vi "Look up Running Measurement Queue .vi"(7 "error in (no error)":errorcluster, 9 "Measurement Name.Harware()":string, 10 "Mag Lab Measure Controller in":refnum<class "Mag Lab Measure Controller.lvclass">) -> (0 "error out":errorcluster, 1 "Measurement Queue":refnum<class "Message Enqueuer.lvclass">, 2 "Found?":bool, 3 "Mag Lab Measure Controller out":refnum<class "Mag Lab Measure Controller.lvclass">)   [LabVIEW 2015, in "Mag Lab Measure Controller.lvclass"]
uses:
  Mag Lab Measure Controller.lvclass
  <vilib>/ActorFramework/Message Enqueuer/Message Enqueuer.lvclass
  Mag Lab Measure Controller.lvclass/Mag Lab Measure Controller.ctl
panel:
  in  "Self Enqueuer":refnum<class "Message Enqueuer.lvclass">
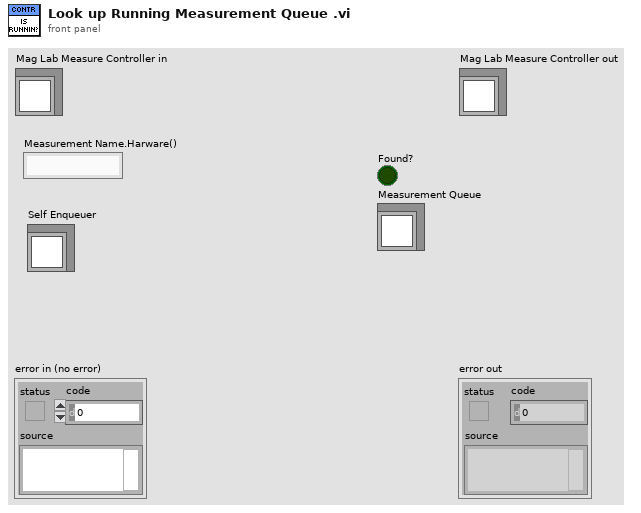
[diagram p1: front panel]
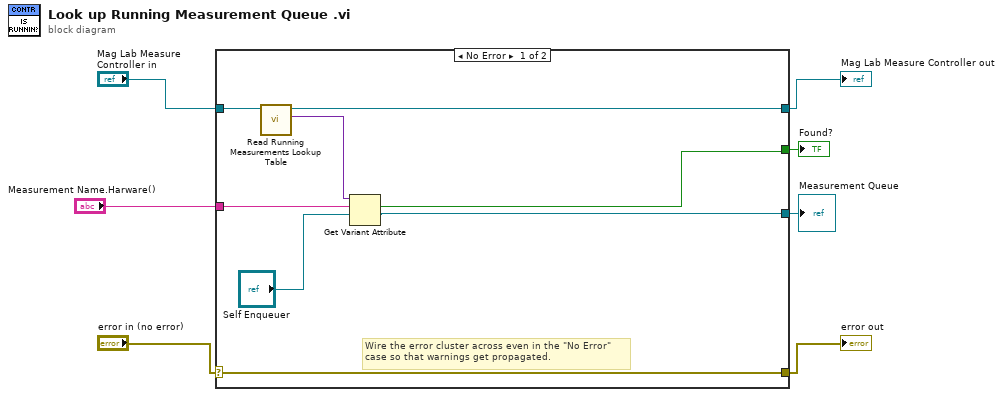
[diagram p0: block diagram]
diagram:
  n1 = case shown="No Error" "error in (no error)" {
    selector: "error in (no error)" -> [w15 w17]
    tunnel: [w15 w17] -> w1
    tunnel: [w11 w16] -> w3
    tunnel: "Mag Lab Measure Controller in" -> [w12 w16]
    tunnel: "Measurement Name.Harware()" -> [w13 _]
    tunnel: [w10 _] -> w5
    tunnel: [w9 _] -> w6
    frame No Error {
      # "Wire the error cluster across even in the \"No Error\"\ncase so that warnings get propagated."
      n2 = call "Read Running Measurements Lookup Table.vi"("Mag Lab Measure Controller in"=w12) -> ("Running Measurements Queue Lookup Table"=w14:variant, "Mag Lab Measure Controller out"=w11:refnum<class "Mag Lab Measure Controller.lvclass">)  [unwired: 8 in, 1 out]
      n3 = Get Variant Attribute(Variant=w14, name=w13, default value (empty Variant)="Self Enqueuer") -> (found=w9:bool, value=w10:refnum<class "Message Enqueuer.lvclass">)  [unwired: 1 in, 2 out]
    }
    frame Error {
    }
  }
  "error out" <- w1
  "Mag Lab Measure Controller out" <- w3
  "Found?" <- w6
  "Measurement Queue" <- w5
